vi "api_mqttSubscribe.vi"(0 "subscriptionInfo":T1[](array[typedef])=[{"Topic"="a/b", "QoS"=enum."At least once"}], 9 "messageID":u16, 11 "error in (no error)":errorcluster) -> (4 "success":bool, 15 "error out":errorcluster)   [LabVIEW 2021, in "mqtt.lvclass"]
uses:
  mqtt.lvclass
  mqttTypedef/mqttSubscribeCluster.ctl
  Control 1.ctl
  mqttTypedef/mqttMessageType.ctl
  mqttCmd/mqttCmdSubscribe/mqttCmdSubscribe.lvclass
  C:/Users/Fujitsu/Desktop/Nouveau dossier/avril/Project mqtt/Src/class/mqtt/mqttCmd/mqttCmd.lvclass
  mqttTypedef/mqttQOSlevel.ctl
  mqttCmd/mqttCmdSubscribe/mqttCmdSubscribe.lvclass/mqttCmdSubscribe.ctl
  mqttCmd/mqttCmd.lvclass/mqttCmd.ctl
  mqttCmd/mqttCmd.lvclass
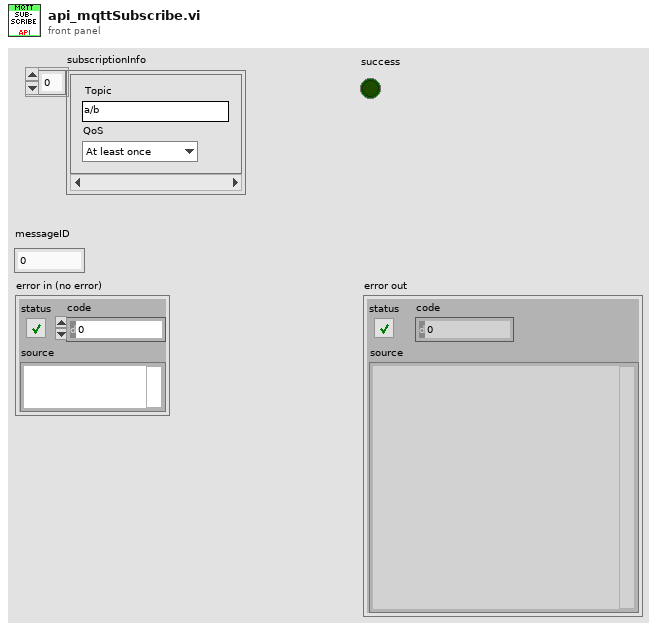
[diagram p1: front panel]
types:
  T1 = typedef "mqttSubscribeCluster.ctl" = cluster{"Topic":T2, "QoS":enum8{"At most once", "At least once", "Exactly once", "Reserved"}}
  T2 = typedef "Control 1.ctl" = string
  T3 = typedef "mqttQOSlevel.ctl" = enum8{"At most once", "At least once", "Exactly once", "Reserved"}
  T4 = typedef "mqttMessageType.ctl" = enum32{"Reserved", "CONNECT", "CONNACK", "PUBLISH", "PUBACK", "PUBREC", "PUBREL", "PUBCOMP", "SUBSCRIBE", "SUBACK", "UNSUBSCRIBE", "UNSUBACK", "PINGREQ", "PINGRESP", "DISCONNECT", "Reserved2"}
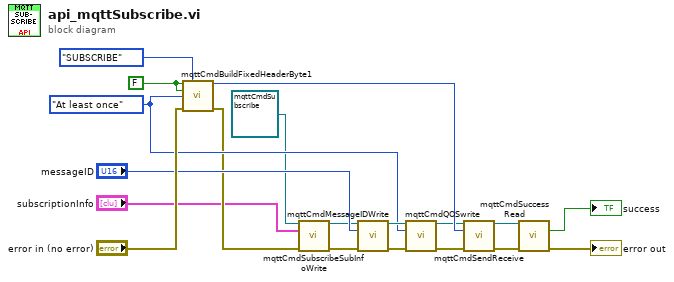
[diagram p0: block diagram]
diagram:
  w7 = mqttQOSlevel."At least once" ("QoS (At most once)")
  w1 = FALSE ("retain(F)")
  n1 = call "mqttCmdBuildFixedHeaderByte1.vi"("retain(F)"=w1, "MessageType"=mqttMessageType."SUBSCRIBE", "duplicate(F)"=w1, "QoS (At most once)"=w7, "error in (no error)"="error in (no error)") -> ("byte1"=w18:u8, "error out"=w6:errorcluster)  [unwired: 9 in]
  n2 = call "mqttCmdSubscribeSubInfoWrite.vi"("mqttSubscribe in"=refnum<class "mqttCmdSubscribe.lvclass"> refnum ("mqttSubscribe.lvclass"), "subscriptionInfo"="subscriptionInfo", "error in (no error)"=w6) -> ("mqttSubscribe out"=w4:refnum<class "mqttCmdSubscribe.lvclass">, "error out"=w5:errorcluster)  [unwired: 11 in]
  n3 = call "mqttCmdMessageIDWrite.vi"("mqttBrokerCommand in"=w4, "messageID"="messageID", "error in (no error)"=w5) -> ("mqttBrokerCommand out"=w9:refnum<class "mqttCmdSubscribe.lvclass">, "error out"=w11:errorcluster)  [unwired: 11 in]
  n4 = call "mqttCmdQOSwrite.vi"("mqttBrokerCommand in"=w9, "QoS"=w7, "error in (no error)"=w11) -> ("mqttBrokerCommand out"=w8:refnum<class "mqttCmdSubscribe.lvclass">, "error out"=w10:errorcluster)  [unwired: 11 in]
  n5 = call "mqttCmdSendReceive.vi"("mqttConnect in"=w8, "byte1"=w18, "error in (no error)"=w10) -> ("mqttConnect out"=w15:refnum<class "mqttCmdSubscribe.lvclass">, "error out"=w16:errorcluster)  [unwired: 10 in, 1 out]
  n6 = call "mqttCmdSuccessRead.vi"("mqttBrokerCommand in"=w15, "error in (no error)"=w16) -> ("success"=→"success":bool, "error out"=→"error out":errorcluster)  [unwired: 11 in, 1 out]
